vi "Twist3d_GetAll.vi"(11 "Twist3d":T1) -> (0 "rX":dbl, 1 "dZ":dbl, 2 "dY":dbl, 3 "dX":dbl, 4 "rY":dbl, 6 "rZ":dbl)   [LabVIEW 2019, in "Trajectory_Library.lvlib"]
doc: "Get the individual components of the TWIST3D data structure\n\nParameters:\n - in twist3D -- TWIST3D data structure\n\nReturns:\n - dx - Linear \"dx\" component.\n - dy - Linear \"dy\" component.\n - dz - Linear \"dz\" component.\n - rx -- Rotation vector x component (radians)\n - ry -- Rotation vector y component (radians)\n - rz -- Rotation vector z component (radians)"
uses:
  Trajectory_Library.lvlib
  TWIST3D.ctl
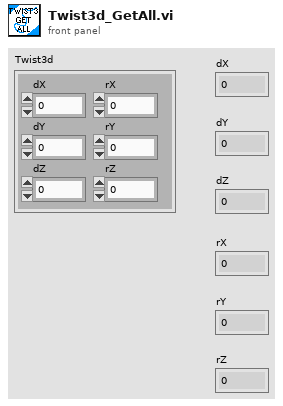
[diagram p1: front panel]
types:
  T1 = typedef "Trajectory_Library.lvlib/TWIST3D.ctl" = cluster{"dX":dbl, "dY":dbl, "dZ":dbl, "rX":dbl, "rY":dbl, "rZ":dbl}
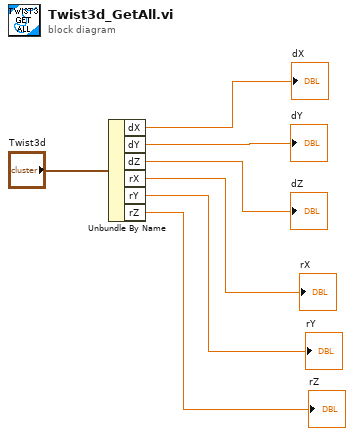
[diagram p0: block diagram]
diagram:
  n1 = Unbundle By Name("Twist3d") -> ("dX"=→"dX":dbl, "dY"=→"dY":dbl, "dZ"=→"dZ":dbl, "rX"=→"rX":dbl, "rY"=→"rY":dbl, "rZ"=→"rZ":dbl)
